vi "GetPltColTable.vi"(8 "ErrorIn(No Error)":errorcluster caption="entrée d'erreur (pas d'erreur)") -> (0 "sortie d'erreur":errorcluster, 3 "Color Table":u32[](array[colorbox]))   [LabVIEW 2012]
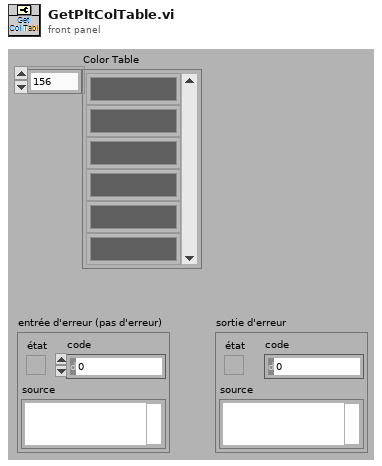
[diagram p1: front panel]
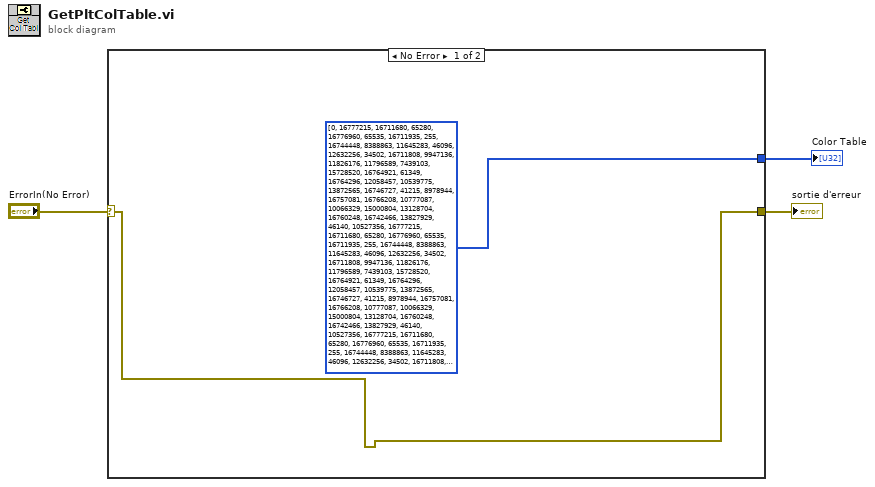
[diagram p0: block diagram]
diagram:
  n1 = case shown="No Error" "ErrorIn(No Error)" {
    selector: "ErrorIn(No Error)" -> [w4 w6]
    tunnel: [w4 w6] -> w2
    tunnel: [u32[] [0, 16777215, 16711680, 65280, 16776960, 65535, 16711935, 255, 16744448, 8388863, 11645283, 46096, 12632256, 34502, 16711808, 9947136, 11826176, 11796589, 7439103, 15728520, 16764921, 61349, 16764296, 12058457, 10539775, 13872565, 16746727, 41215, 8978944, 16757081, 16766208, 10777087, 10066329, 15000804, 13128704, 16760248, 16742466, 13827929, 46140, 10527356, 16777215, 16711680, 65280, 16776960, 65535, 16711935, 255, 16744448, 8388863, 11645283, 46096, 12632256, 34502, 16711808, 9947136, 11826176, 11796589, 7439103, 15728520, 16764921, 61349, 16764296, 12058457, 10539775, 13872565, 16746727, 41215, 8978944, 16757081, 16766208, 10777087, 10066329, 15000804, 13128704, 16760248, 16742466, 13827929, 46140, 10527356, 16777215, 16711680, 65280, 16776960, 65535, 16711935, 255, 16744448, 8388863, 11645283, 46096, 12632256, 34502, 16711808, 9947136, 11826176, 11796589, 7439103, 15728520, 16764921, 61349, 16764296, 12058457, 10539775, 13872565, 16746727, 41215, 8978944, 16757081, 16766208, 10777087, 10066329, 15000804, 13128704, 16760248, 16742466, 13827929, 46140, 10527356, 16777215, 16711680, 65280, 16776960, 65535, 16711935, 255, 16744448, 8388863, 11645283, 46096, 12632256, 34502, 16711808, 9947136, 11826176, 11796589, 7439103, 15728520, 16764921, 61349, 16764296, 12058457, 10539775, 13872565, 16746727, 41215, 8978944, 16757081, 16766208, 10777087, 10066329, 15000804, 13128704, 16760248, 16742466, 13827929, 46140, 10527356] ("tableau") _] -> w1
    frame No Error {
    }
    frame Error {
    }
  }
  "sortie d'erreur" <- w2
  "Color Table" <- w1
